vi "Get Attribute - Array.vi"(8 "error in (no error)":errorcluster, 10 "Key":string, 11 "YAML Parser in":refnum<class "YAML Parser.lvclass">) -> (0 "error out":errorcluster, 1 "Is Null?":bool, 2 "Array":refnum<class "YAML Parser.lvclass">, 3 "YAML Parser out":refnum<class "YAML Parser.lvclass">)   [LabVIEW 2015, in "YAML Parser.lvclass"]
uses:
  YAML Parser.lvclass
  YAML Parser.lvclass/YAML Parser.ctl
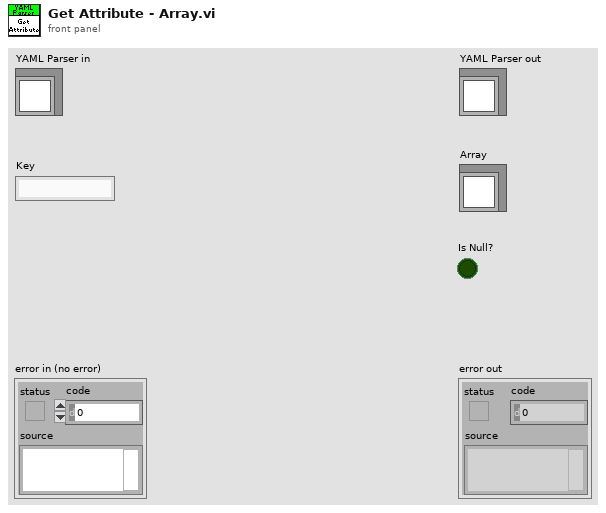
[diagram p1: front panel]
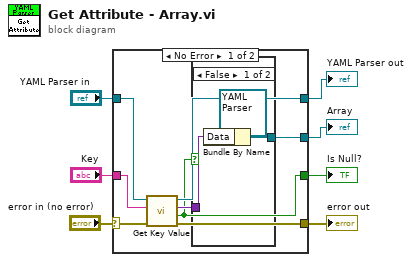
[diagram p0: block diagram]
diagram:
  n1 = case shown="No Error" "error in (no error)" {
    selector: "error in (no error)" -> [w15 w20]
    tunnel: [w14 w20] -> w6
    tunnel: [w12 w19] -> w4
    tunnel: "YAML Parser in" -> [w13 w19]
    tunnel: "Key" -> [w11 _]
    tunnel: [w9 _] -> w2
    tunnel: [w8 _] -> w1
    frame No Error {
      n2 = call "Get Key Value.vi"("error in (no error)"=w15, "Key"=w11, "YAML Parser in"=w13) -> ("error out"=w14:errorcluster, "Is Null?"=w9:bool, "Key Value"=w10:variant, "YAML Parser out"=w12:refnum<class "YAML Parser.lvclass">)  [unwired: 5 in]
      n3 = case shown="False" w9 {
        tunnel: w10 -> [w17 _]
        tunnel: [w16 _] -> w8
        frame False {
          n4 = Bundle By Name(cluster=refnum<class "YAML Parser.lvclass"> refnum ("Array"), "Data"=w17) -> (w16:refnum<class "YAML Parser.lvclass">)
        }
        frame True {
        }
      }
    }
    frame Error {
    }
  }
  "error out" <- w6
  "YAML Parser out" <- w4
  "Is Null?" <- w2
  "Array" <- w1
